vi "Actor Core.vi"(8 "error in":errorcluster, 11 "Channel Selector in":refnum<class "Devices to Load.lvclass">) -> (0 "error out":errorcluster, 3 "Actor out":refnum<class "Actor.lvclass">)   [LabVIEW 2018, in "Devices to Load Config Actor.lvlib" / "Devices to Load.lvclass"]
doc: "(<B>Filename</B>: Actor Framework.lvlib:Actor.lvclass:Actor Core.vi)\n\nReceives messages to the actor, reacts to them, and initiates any error handling that may shut the actor down.\n\nDescendant classes may override this VI to append parallel tasks for the actor to complete while it handles messages. Overrides use the Call Parent Method node."
uses:
  Devices to Load.lvclass
  C:/Program Files (x86)/National Instruments/LabVIEW 2018/vi.lib/ActorFramework/Actor/Actor.lvclass
  <vilib>/ActorFramework/Actor/Actor.lvclass
  Devices to Load.lvclass/Devices to Load.ctl
  <vilib>/ActorFramework/Actor/Actor.lvclass/Actor.ctl
  <vilib>/ActorFramework/Message Enqueuer/Message Enqueuer.lvclass/Message Enqueuer.ctl
  Devices to Load Messages/Return Devices to Load IDs Msg/Return Devices to Load IDs Msg.lvclass/Return Devices to Load IDs Msg.ctl
  <vilib>/ActorFramework/Message Enqueuer/Init from Existing Queue.vi
  <vilib>/ActorFramework/Message Enqueuer/Enqueue.vi
  <vilib>/ActorFramework/Stop Msg/Stop Msg.lvclass
  C:/Program Files (x86)/National Instruments/LabVIEW 2018/vi.lib/ActorFramework/Message/Message.lvclass
  Devices to Load Messages/Return Devices to Load IDs Msg/Return Devices to Load IDs Msg.lvclass
  <vilib>/ActorFramework/Message Priority Queue/Priority Enqueue.vi
  <vilib>/ActorFramework/Message Enqueuer/Message Enqueuer.lvclass
panel:
  in  "Microgrid ID":u8=1 min=1 max=232 step=1
  in  "Cancel Button":bool
  in  "OK Button":bool
  in  "Channels":i32[](listbox)
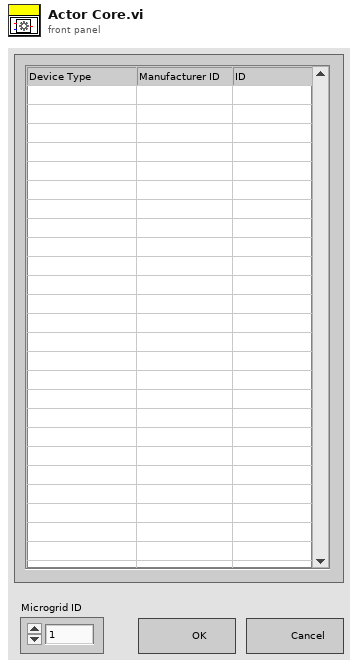
[diagram p1: front panel]
types:
  T1 = enum32{"Invalid", "Standard", "Closed", "Hidden", "Minimized", "Maximized"}
  T2 = typedef "Devices to Load Config Actor.lvlib/Devices to Load.lvclass/Devices to Load User Events.ctl" = cluster{"ItemNames":refnum<user-event>, "stop":refnum<user-event>}
  T3 = typedef "CSEISMIC DDS.lvlib/CSEISMIC DDS.lvclass/DeviceID.ctl" = string
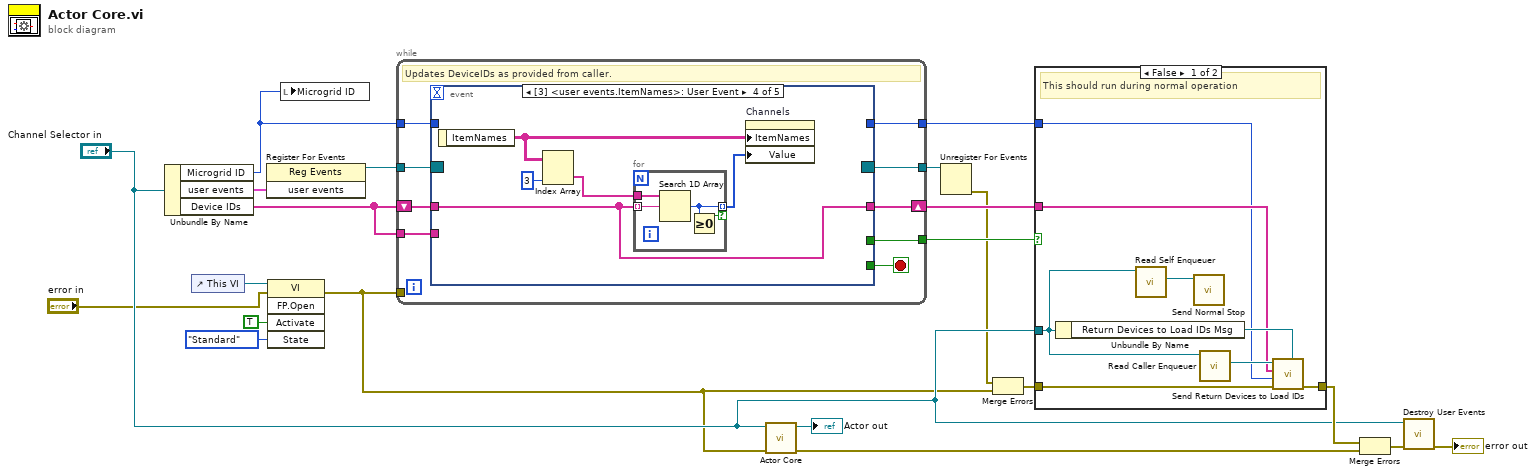
[diagram p0: block diagram]
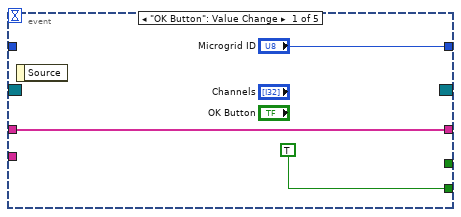
[diagram p3: hidden frame]
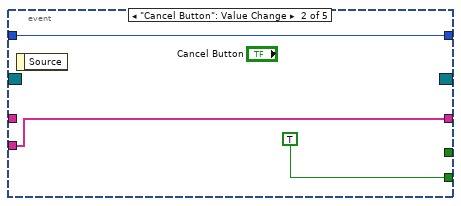
[diagram p4: hidden frame]
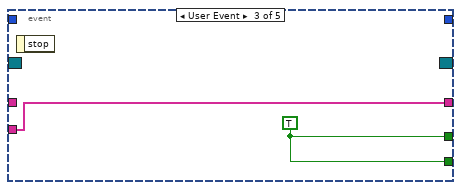
[diagram p5: hidden frame]
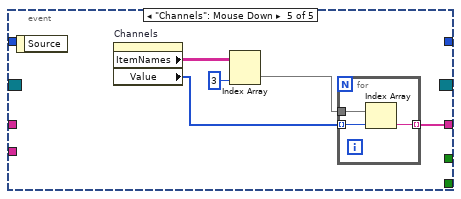
[diagram p6: hidden frame]
diagram:
  n1 = Unbundle By Name("Channel Selector in") -> ("Microgrid ID"=w6:u8, "user events"=w18:T2, "Device IDs"=w16:T3[])
  n2 = control-ref of="This VI"() -> (w5:refnum<vi>)
  n3 = register-events(w18) -> (reference out=w17:refnum<event-registration>)  [unwired: 2 in, 1 out]
  n4 = invoke class="VI" method="FP.Open"(reference=w5, error in="error in", "Activate"=TRUE ("Activate?"), "State"=T1."Standard") -> (error out=w1:errorcluster)  [unwired: 1 in, 4 out]
  n5 = local write "Microgrid ID"(w6) -> ()
  n6 = while {
    tunnel: w17 -> [w28]
    shift-right: [w27] -> w15
    shift-left: w16 -> [w29]
    tunnel: w16 -> [w26]
    tunnel: [w25] -> w14
    tunnel: [w24] -> w11
    tunnel: w6 -> [w23]
    tunnel: [w22] -> w7
    tunnel: w1 -> [_]
    stop <- w30 stop-if-true
    # "Updates DeviceIDs as provided from caller."
    n7 = event shown="[3] <user events.ItemNames>: User Event" {
      selector: w28 -> [_ _ _ _ _]
      dyn-events: [_ _ _ _ _] -> w25
      timeout: _ -> [_ _ _ _ _]
      tunnel: [TRUE TRUE w37 _ _] -> w30
      tunnel: w29 -> [w32 _ _ w40 _]
      tunnel: [w32 w35 w38 w40 w49] -> w27
      tunnel: w26 -> [_ w35 w38 _ _]
      tunnel: [_ _ w37 _ _] -> w24
      tunnel: w23 -> [_ w34 _ _ _]
      tunnel: ["Microgrid ID" w34 _ _ _] -> w22
      event "OK Button": Value Change {
        n8 = event-data() -> ()  [unwired: 1 in, 1 out]
      }
      event "Cancel Button": Value Change {
        n9 = event-data() -> ()  [unwired: 1 in, 1 out]
      }
      event User Event {
        w37 = TRUE
        n10 = event-data() -> ()  [unwired: 1 in, 1 out]
      }
      event User Event {
        n11 = event-data() -> ("ItemNames"=w42:string[][])  [unwired: 1 in]
        n12 = Index Array(array=w42, index (col)=3 ("disabled index (col)")) -> (element=w39:string[])  [unwired: 1 in]
        n13 = for {
          tunnel: w39 -> [w47]
          tunnel: w40 -> [w46] mode=indexing
          tunnel: [w45] -> w41 mode=indexing if=w44
          n14 = Search 1D Array(1D array=w47, element=w46) -> (index of element=w45:i32)  [unwired: 1 in]
          n15 = Greater Or Equal To 0?(x=w45) -> (x >= 0?=w44:bool)
        }
        n16 = property on="Channels" class="MCListbox (strict)"("ItemNames"=w42, "Value"=w41) -> ()  [unwired: 2 in, 2 out]
      }
      event "Channels": Mouse Down {
        n17 = event-data() -> ()  [unwired: 1 in, 1 out]
        n18 = property on="Channels" class="MCListbox (strict)"() -> ("ItemNames"=w51:string[][], "Value"=w50:i32[])  [unwired: 2 in, 2 out]
        n19 = Index Array(array=w51, index (col)=3 ("disabled index (col)")) -> (element=w48:string[])  [unwired: 1 in]
        n20 = for {
          tunnel: w50 -> [w54] mode=indexing
          tunnel: w48 -> [w55]
          tunnel: [w53] -> w49 mode=indexing
          n21 = Index Array(array=w55, index=w54) -> (element=w53:string)
        }
      }
    }
  }
  n22 = call-parent "Actor Core.vi"("error in"=w1, "Actor in"="Channel Selector in") -> ("error out"=w21:errorcluster, "Actor out"=→"Actor out":refnum<class "Actor.lvclass">)  [unwired: 8 in]
  n23 = Unregister For Events(event registration refnum=w14) -> (error out=w8:errorcluster)  [unwired: 1 in]
  n24 = Merge Errors(w8, w1) -> (w9:errorcluster)
  n25 = case shown="False" w11 {
    tunnel: [w57 w64] -> w19
    tunnel: w9 -> [w60 w64]
    tunnel: w15 -> [w59 _]
    tunnel: "Channel Selector in" -> [w58 _]
    tunnel: w7 -> [w56 _]
    frame False {
      # "This should run during normal operation"
      n26 = Unbundle By Name(w58) -> ("Return Devices to Load IDs Msg"=w63:refnum<class "Return Devices to Load IDs Msg.lvclass">)
      n27 = call <vilib>:"Read Self Enqueuer.vi"("Actor"=w58) -> ("Self Enqueuer"=w61:refnum<class "Message Enqueuer.lvclass">)  [unwired: 10 in]
      n28 = call <vilib>:"Send Normal Stop.vi"("Message Enqueuer"=w61) -> ()  [unwired: 10 in, 1 out]
      n29 = call <vilib>:"Read Caller Enqueuer.vi"("Actor"=w58) -> ("Caller Enqueuer"=w62:refnum<class "Message Enqueuer.lvclass">)  [unwired: 10 in]
      n30 = call "Send Return Devices to Load IDs.vi"("Message Type"=w63, "error in (no error)"=w60, "Microgrid ID"=w56, "Device IDs"=w59, "Message Enqueuer"=w62) -> ("error out"=w57:errorcluster)  [unwired: 5 in, 1 out]
    }
    frame True {
      # "This executes when the actor is stopped programmatically rather than through the UI."
    }
  }
  n31 = Merge Errors(w19, w21) -> (w13:errorcluster)
  n32 = call "Destroy User Events.vi"("error in"=w13, "Devices to Load in"="Channel Selector in") -> ("error out"=→"error out":errorcluster)  [unwired: 8 in, 1 out]
